vi "get full path of target vi.vi"(8 "class folder path":path, 9 "class vi names":string[](array[string]), 10 "class vi paths":path[](array[path]), 11 "vi to qualify":string) -> (2 "not in class":bool, 3 "full path":path)   [LabVIEW 2013]
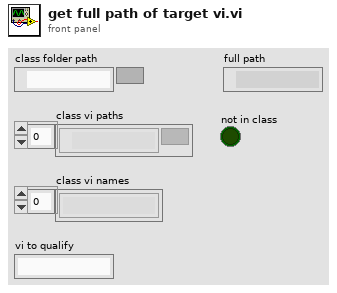
[diagram p1: front panel]
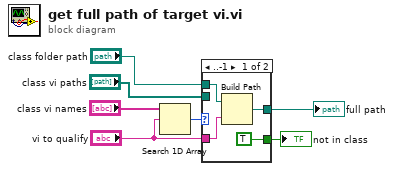
[diagram p0: block diagram]
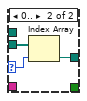
[diagram p2: hidden frame]
diagram:
  n1 = Search 1D Array(1D array="class vi names", element="vi to qualify") -> (index of element=w2:i32)  [unwired: 1 in]
  n2 = case shown="..-1" w2 {
    selector: w2 -> [_ w13]
    tunnel: "class vi paths" -> [_ w14]
    tunnel: [w9 w12] -> w7
    tunnel: "vi to qualify" -> [w11 _]
    tunnel: "class folder path" -> [w10 _]
    tunnel: [TRUE _] -> w1
    frame ..-1 {
      n3 = Build Path(base path=w10, name or relative path=w11) -> (appended path=w9:path)
    }
    frame 0.. {
      n4 = Index Array(array=w14, index=w13) -> (element=w12:path)
    }
  }
  "full path" <- w7
  "not in class" <- w1
